vi "CreateQueue.vi"(8 "Error In":errorcluster, 9 "Max Queue Size":i32=-1) -> (0 "Error Out":errorcluster, 1 "Trace Out":refnum<queue>)   [LabVIEW 2018, in "TracerLibrary.lvlib" / "Tracer.lvclass"]
uses:
  Tracer.lvclass
  protected/Tracer_ClassAttributes.vi
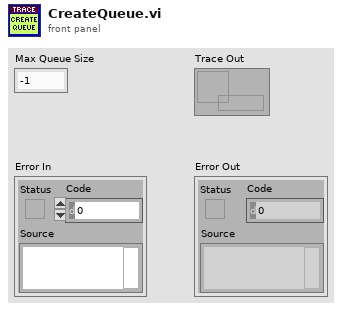
[diagram p1: front panel]
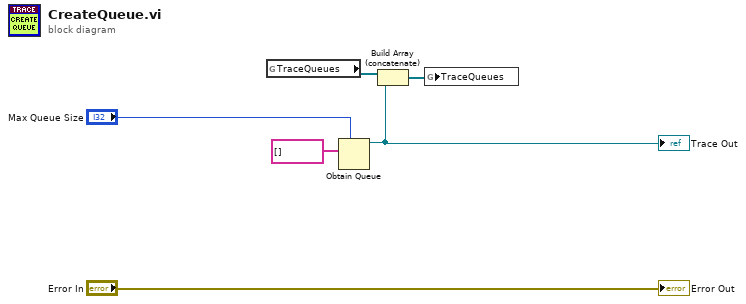
[diagram p0: block diagram]
diagram:
  n1 = global read "Tracer_ClassAttributes.vi" "TraceQueues"() -> (w2:refnum<queue>[])
  n2 = Obtain Queue(max queue size (-1, unlimited)="Max Queue Size", element data type=string[] []) -> (queue out=w4:refnum<queue>)  [unwired: 3 in, 2 out]
  "Trace Out" <- w4
  n3 = Build Array (concatenate)(w2, w4) -> (w1:refnum<queue>[])
  n4 = global write "Tracer_ClassAttributes.vi" "TraceQueues"(w1) -> ()
  "Error Out" <- "Error In"
